vi "Create DI Mode.vi"(7 "mode settings":variant, 8 "error in":errorcluster, 9 "number of channels":i32, 10 "channel settings":T1[](array[typedef]), 11 "digital input mode in":refnum<class "Digital Input Mode.lvclass">) -> (0 "error out":errorcluster, 1 "channels":refnum<class "Channel.lvclass">[](array[class]), 3 "digital input mode out":refnum<class "Digital Input Mode.lvclass">)   [LabVIEW 2017, in "Scan Engine Scripting.lvlib" / "Digital Input Mode.lvclass"]
uses:
  Digital Input Mode.lvclass
  Channel Classes/Channel/Channel.lvclass
  Controls/digital channel settings.ctl
  Channel Classes/DI Channel/DI Channel.lvclass
  C:/dev/github.com/debryant/niveristand-scan-engine-ethercat-custom-device/Custom Device Source/Scripting/Modules/Channel Classes/Channel/Channel.lvclass
  Scan Engine Scripting.lvlib
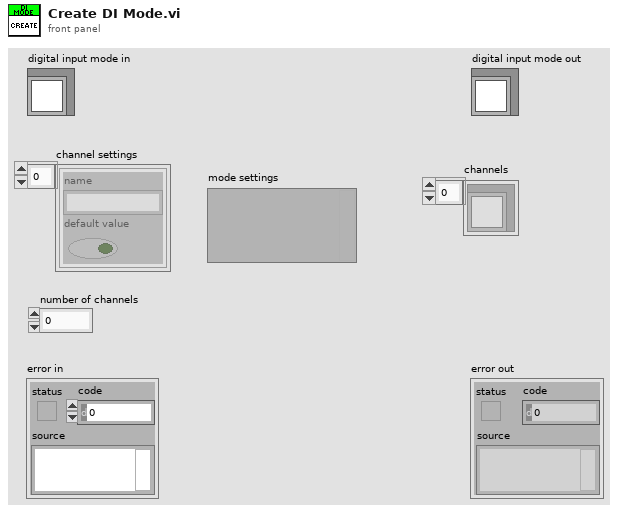
[diagram p1: front panel]
types:
  T1 = typedef "Scan Engine Scripting.lvlib/digital channel settings.ctl" = cluster{"name":string, "default value":bool}
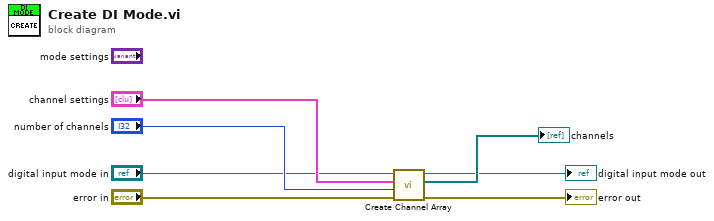
[diagram p0: block diagram]
diagram:
  n1 = call "Create Channel Array.vi"("error in"="error in", "expected channel count"="number of channels", "channel settings"="channel settings", "digital input mode in"="digital input mode in") -> ("error out"=→"error out":errorcluster, "channels"=→"channels":refnum<class "DI Channel.lvclass">[], "digital input mode out"=→"digital input mode out":refnum<class "Digital Input Mode.lvclass">)  [unwired: 5 in]
